vi "TestUnpackFields.vi"() -> ()   [LabVIEW 2019]
uses:
  labview source/gRPC lv Support/Server API/typeDefs/Message Element Type.ctl
  9a6836f9-9a56-4eab-8b5d-32a2dab5a538.vi
  945ff6c4-0d84-4f7a-9a8f-55dc7e3ca4cd.vi
  2615de07-9be7-4ab4-a6b4-9b34c4a81146.vi
  0ef81a5d-c64c-4909-85c0-d19ab57e7b9c.vi
  81517bb0-4ee5-4bad-b694-1fb8e52814d0.vi
  dadd9c8a-ddff-4703-8d6c-89fc272dbf14.vi
  8c3f2268-867d-41bc-b743-d5f3d9e44b17.vi
  e9f3ca52-b107-44b2-9fe7-14ac293a788e.vi
  b0b1f67d-1579-4d00-9960-16947ef342fe.vi
  0bfe02f5-357b-4b4f-92fb-344ae4da9c22.vi
  c675992c-3555-4a6a-92dd-007508fb3f55.vi
  0274b7ac-654e-4932-bfa3-c92a453a9d62.vi
  labview source/gRPC lv Support/Server API/Translate Protobuf Error.vi
  <vilib>/AdvancedString/1D String Array to Delimited String.vi
  labview source/gRPC lv Support/Server API/Server/Get Server DLL Path.vi
  labview source/gRPC lv Support/grpc-lvsupport.lvlib
panel:
  out "value 6":bool
  out "value 5":string
  out "value 4":sgl[](array[numeric])
  out "value 3":dbl
  out "value 2":sgl format="%.8f"
  out "value":i32
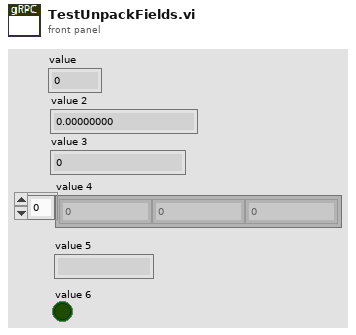
[diagram p1: front panel]
types:
  T1 = typedef "grpc-lvsupport.lvlib/Message Element Type.ctl" = enum32{"Int32Value", "FloatValue", "DoubleValue", "BoolValue", "StringValue", "MessageValue", "Int64Value", "UInt32Value", "UInt64Value", "EnumValue", "Bytes", "Fixed64", "Fixed32", "SFixed64", "SFixed32", "SInt64", "SInt32"}
  T2 = typedef "grpc-lvsupport.lvlib/grpcId.ctl" = u64
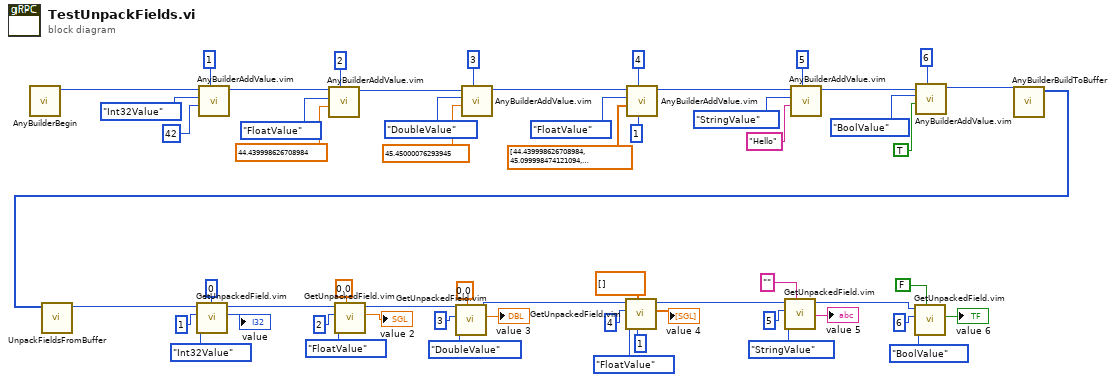
[diagram p0: block diagram]
diagram:
  n1 = call "AnyBuilderBegin.vi"() -> ("Builder Ref Out"=w58:T2)  [unwired: 9 in, 1 out]
  n2 = call "AnyBuilderAddValue.vim"("protobufId"=1, "Value"=42, "MessageElementType"=Message_Element_Type."Int32Value", "gRPCid in"=w58) -> ("gRPCid out"=w47:u64)  [unwired: 6 in, 1 out]
  n3 = call "AnyBuilderAddValue.vim"("protobufId"=2, "Value"=sgl 44.44, "MessageElementType"=Message_Element_Type."FloatValue", "gRPCid in"=w47) -> ("gRPCid out"=w39:u64)  [unwired: 6 in, 1 out]
  n4 = call "AnyBuilderAddValue.vim"("protobufId"=3, "Value"=45.45000076293945, "MessageElementType"=Message_Element_Type."DoubleValue", "gRPCid in"=w39) -> ("gRPCid out"=w30:u64)  [unwired: 6 in, 1 out]
  n5 = call "AnyBuilderAddValue.vim"("isRepeated"=1, "protobufId"=4, "Value"=sgl[] [44.44, 45.1, 46.2], "MessageElementType"=Message_Element_Type."FloatValue", "gRPCid in"=w30) -> ("gRPCid out"=w21:u64)  [unwired: 5 in, 1 out]
  n6 = call "AnyBuilderAddValue.vim"("protobufId"=5, "Value"="Hello", "MessageElementType"=Message_Element_Type."StringValue", "gRPCid in"=w21) -> ("gRPCid out"=w13:u64)  [unwired: 6 in, 1 out]
  n7 = call "AnyBuilderAddValue.vim"("protobufId"=6, "Value"=TRUE, "MessageElementType"=Message_Element_Type."BoolValue", "gRPCid in"=w13) -> ("gRPCid out"=w12:u64)  [unwired: 6 in, 1 out]
  n8 = call "AnyBuilderBuildToBuffer.vi"("Builder Ref"=w12) -> ("Buffer"=w6:u8[])  [unwired: 9 in, 1 out]
  n9 = call "UnpackFieldsFromBuffer.vi"("Buffer"=w6) -> ("Fields Ref Out"=w8:T2)  [unwired: 9 in, 1 out]
  n10 = call "GetUnpackedField.vim"("Value"=0, "MessageElementType"=Message_Element_Type."Int32Value", "protobufId"=1, "gRPCid in"=w8) -> ("value"=→"value":i32, "gRPCid out"=w5:u64)  [unwired: 5 in, 1 out]
  n11 = call "GetUnpackedField.vim"("Value"=sgl 0.0, "MessageElementType"=Message_Element_Type."FloatValue", "protobufId"=2, "gRPCid in"=w5) -> ("value"=→"value 2":sgl, "gRPCid out"=w1:u64)  [unwired: 5 in, 1 out]
  n12 = call "GetUnpackedField.vim"("Value"=0.0, "MessageElementType"=Message_Element_Type."DoubleValue", "protobufId"=3, "gRPCid in"=w1) -> ("value"=→"value 3":dbl, "gRPCid out"=w4:u64)  [unwired: 5 in, 1 out]
  n13 = call "GetUnpackedField.vim"("isRepeated"=1, "Value"=sgl[] [], "MessageElementType"=Message_Element_Type."FloatValue", "protobufId"=4, "gRPCid in"=w4) -> ("value"=→"value 4":sgl[], "gRPCid out"=w3:u64)  [unwired: 4 in, 1 out]
  n14 = call "GetUnpackedField.vim"("Value"="", "MessageElementType"=Message_Element_Type."StringValue", "protobufId"=5, "gRPCid in"=w3) -> ("value"=→"value 5":string, "gRPCid out"=w2:u64)  [unwired: 5 in, 1 out]
  n15 = call "GetUnpackedField.vim"("Value"=FALSE, "MessageElementType"=Message_Element_Type."BoolValue", "protobufId"=6, "gRPCid in"=w2) -> ("value"=→"value 6":bool)  [unwired: 5 in, 2 out]
